vi "PH_BL-Master.Set Objects RC.vi"(0 "VI in":refnum<vi>, 1 "Boolean Status Service Subscriber before":T4(array[cluster]) {"Status" items=["no info", "off/false/out", "on/true/in", "Failure", "Alarm", "Status 1", "Status 2", "Status 3"]}, 2 "Picture Status Service Subscriber before":T4(array[cluster]) {"Status" items=["no info", "off/false/out", "on/true/in", "Failure", "Alarm", "Status 1", "Status 2", "Status 3"]}, 3 "Vacua before":T1(array[cluster]), 5 "error in (no error)":errorcluster) -> (14 "VI out":refnum<vi>, 19 "error out":errorcluster)   [LabVIEW 2014, in "PH_BL-Master.lvlib"]
uses:
  PH_BL-Master.lvlib
  PH_StatusHandler/PH_StatusHandler.Status.ctl
  PH_BL-Master.Status Subscriber Class.ctl
  PH_VacuumControl/PH_VacuumControl.lvlib
  PH_Common/PH_Common.lvlib
  PH_StatusHandler/PH_StatusHandler.lvlib
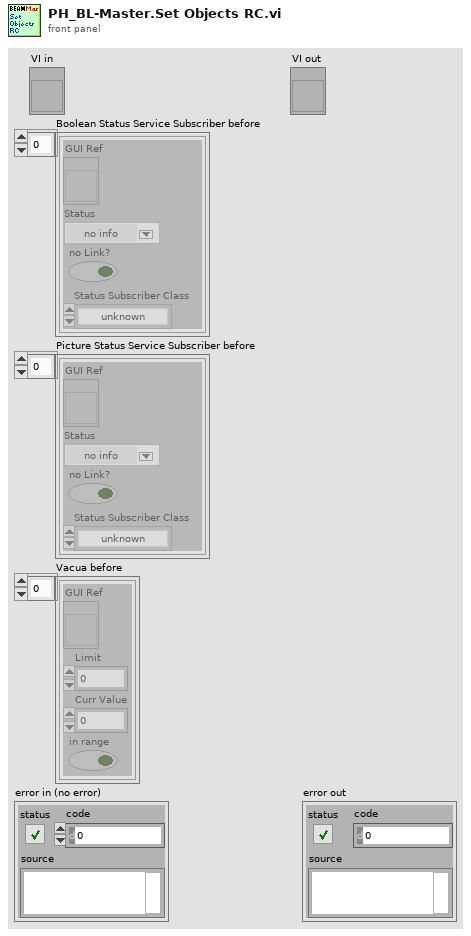
[diagram p1: front panel]
types:
  T1 = cluster{"GUI Ref":refnum<vi>, "Limit":dbl, "Curr Value":dbl, "in range":bool}[]
  T2 = typedef "PH_StatusHandler.lvlib/PH_StatusHandler.Status.ctl" = i16
  T3 = typedef "PH_BL-Master.lvlib/PH_BL-Master.Status Subscriber Class.ctl" = enum16{"unknown", "Switch", "BB", "6P Switch", "Switch GUI", "Switch and 6P State", "Force Sensor"}
  T4 = cluster{"GUI Ref":refnum<vi>, "Status":T2, "no Link?":bool, "Status Subscriber Class":T3}[]
  T5 = typedef "PH_BL-Master.lvlib/PH_BL-Master.i attribute.ctl" = cluster{"Remote controlled":bool, "Boolean Condition Service Subscriber":refnum<vi>[], "Picture Condition Service Subscriber":refnum<vi>[], "R2S":cluster{"GUI Ref":refnum<vi>, "State":bool}, "Vacua":cluster{"GUI Ref":refnum<vi>, "Limit":dbl, "Curr Value":dbl, "in range":bool}[], "O2 Inspection":cluster{"GUI Ref":refnum<vi>, "Concentration":dbl, "State":T2}[], "Boolean Status Service Subscriber":cluster{"GUI Ref":refnum<vi>, "Status":T2, "no Link?":bool, "Status Subscriber Class":T3}[], "Picture Status Service Subscriber":cluster{"GUI Ref":refnum<vi>, "Status":T2, "no Link?":bool, "Status Subscriber Class":T3}[], "6P 4Q Service Subscriber":cluster{"GUI Ref":refnum<vi>, "Selector":T6, "no Link?":bool}[], "Index of latest 6P 4Q changing Instance":i32, "Index of latest Picture Status changing Instance":i32, "Index of latest Boolean Status changing Instance":i32, "Vision ID on same Node":string, "Start Phase over?":bool, "GUI Ref Delete":refnum<vi>}
  T6 = typedef "PH_4_Pos_Selector.lvlib/PH_4_Pos_Selector.Position Selector.ctl" = u16
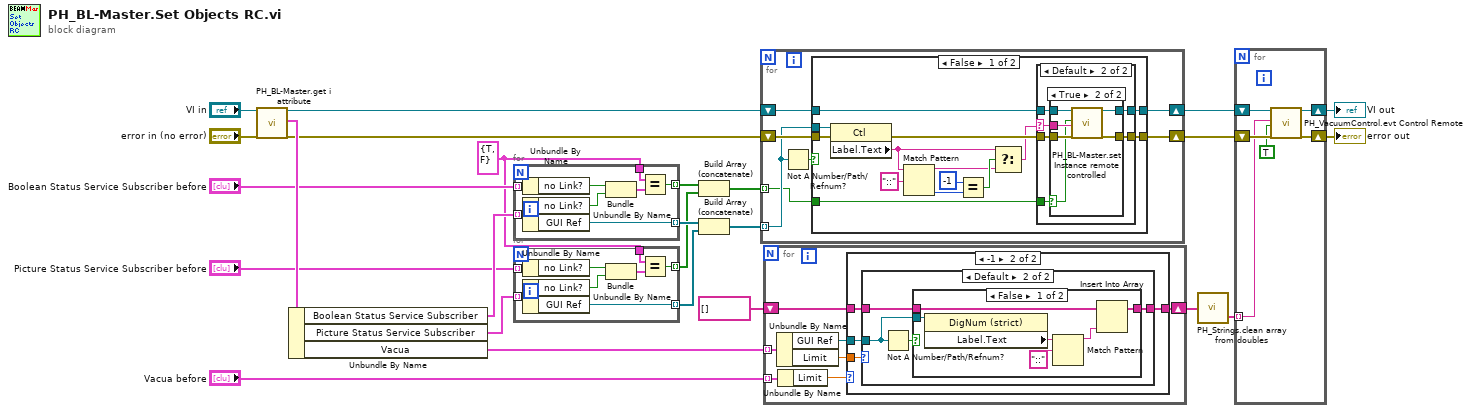
[diagram p0: block diagram]
diagram:
  w6 = cluster{"linked?":bool, "linked?":bool} {"linked?"=TRUE, "linked?"=FALSE} ("x")
  n1 = call "PH_BL-Master.get i attribute.vi"("i ref in"="VI in", "error in (no error)"="error in (no error)") -> ("i ref out"=w17:refnum<vi>, "i attribute"=w20:T5, "error out"=w19:errorcluster)  [unwired: 15 in]
  n2 = Unbundle By Name(w20) -> ("Boolean Status Service Subscriber"=w9:T4, "Picture Status Service Subscriber"=w2:T4, "Vacua"=w14:T1)
  n3 = for {
    tunnel: w9 -> [w33] mode=indexing
    tunnel: [w26] -> w8 mode=indexing
    tunnel: "Boolean Status Service Subscriber before" -> [w32] mode=indexing
    tunnel: w6 -> [w28]
    tunnel: [w27] -> w7 mode=indexing
    n4 = Unbundle By Name(w32) -> ("no Link?"=w31:bool)
    n5 = Unbundle By Name(w33) -> ("no Link?"=w30:bool, "GUI Ref"=w26:refnum<vi>)
    n6 = Bundle("no Link?"=w31, "no Link?"=w30) -> (w29:cluster{"no Link?":bool, "no Link?":bool})  [unwired: 1 in]
    n7 = Equal?(x=w28, y=w29) -> (x = y?=w27:bool)
  }
  n8 = for {
    tunnel: w2 -> [w41] mode=indexing
    tunnel: [w34] -> w5 mode=indexing
    tunnel: "Picture Status Service Subscriber before" -> [w40] mode=indexing
    tunnel: w6 -> [w36]
    tunnel: [w35] -> w4 mode=indexing
    n9 = Unbundle By Name(w40) -> ("no Link?"=w39:bool)
    n10 = Unbundle By Name(w41) -> ("no Link?"=w38:bool, "GUI Ref"=w34:refnum<vi>)
    n11 = Bundle("no Link?"=w39, "no Link?"=w38) -> (w37:cluster{"no Link?":bool, "no Link?":bool})  [unwired: 1 in]
    n12 = Equal?(x=w36, y=w37) -> (x = y?=w35:bool)
  }
  n13 = Build Array (concatenate)(w7, w4) -> (w11:bool[])
  n14 = Build Array (concatenate)(w8, w5) -> (w15:refnum<vi>[])
  n15 = for {
    shift-right: [w46] -> w21
    shift-left: w17 -> [w47]
    shift-right: [w45] -> w22
    shift-left: w19 -> [w48]
    tunnel: w15 -> [w43] mode=indexing
    tunnel: w11 -> [w42] mode=indexing
    n16 = Not A Number/Path/Refnum?(number/path/refnum=w43) -> (NaN/Path/Refnum?=w44:bool)
    n17 = case shown="False" w44 {
      tunnel: w48 -> [w62 w79]
      tunnel: w47 -> [w61 w80]
      tunnel: [w60 w80] -> w46
      tunnel: [w59 w79] -> w45
      tunnel: w43 -> [w57 _]
      tunnel: w42 -> [w50 _]
      frame False {
        n18 = property class="Ctl"(reference=w57, error in=w62) -> (error out=w58:errorcluster, "Label.Text"=w52:string)  [unwired: 1 out]
        n19 = Match Pattern(string=w52, regular expression="::") -> (before substring=w51:string, offset past match=w55:i32)  [unwired: 1 in, 2 out]
        n20 = Equal?(x=-1, y=w55) -> (x = y?=w53:bool)
        n21 = Select(t=w52, s=w53, f=w51) -> (s? t:f=w49:string)
        n22 = case shown="Default" w49 {
          selector: w49 -> [_ w65]
          tunnel: w61 -> [w64 w70]
          tunnel: [w64 w69] -> w60
          tunnel: [w63 w68] -> w59
          tunnel: w58 -> [w63 w67]
          tunnel: w50 -> [_ w66]
          frame "Shutter_Exp_Laserbay_Interlock", "Shutter_Laserlab_Interlock" {
          }
          frame Default {
            n23 = case shown="True" w66 {
              selector: w66 -> [_ w73]
              tunnel: w67 -> [w71 w78]
              tunnel: w70 -> [w72 w77]
              tunnel: [w72 w76] -> w69
              tunnel: [w71 w75] -> w68
              tunnel: w65 -> [_ w74]
              frame False {
              }
              frame True {
                n24 = call "PH_BL-Master.set Instance remote controlled.vi"("i ref in"=w77, "Remote Controlled (false)"=w73, "Instance Name"=w74, "error in"=w78) -> ("i ref out"=w76:refnum<vi>, "error out"=w75:errorcluster)  [unwired: 14 in]
              }
            }
          }
        }
      }
      frame True {
      }
    }
  }
  n25 = for {
    tunnel: w14 -> [w87] mode=indexing
    shift-right: [w85] -> w23
    shift-left: string[] [] -> [w84]
    tunnel: "Vacua before" -> [w82] mode=indexing
    n26 = Unbundle By Name(w87) -> ("GUI Ref"=w86:refnum<vi>, "Limit"=w83:dbl)
    n27 = Unbundle By Name(w82) -> ("Limit"=w81:dbl)
    n28 = case shown="-1" w81 {
      tunnel: w86 -> [_ w92]
      tunnel: [w88 w91] -> w85
      tunnel: w84 -> [w88 w90]
      tunnel: w83 -> [_ w89]
      frame 0, Default {
      }
      frame -1 {
        n29 = case shown="Default" w89 {
          tunnel: w92 -> [_ w96]
          tunnel: [w93 w95] -> w91
          tunnel: w90 -> [w93 w94]
          frame -1 {
          }
          frame Default {
            n30 = Not A Number/Path/Refnum?(number/path/refnum=w96) -> (NaN/Path/Refnum?=w97:bool)
            n31 = case shown="False" w97 {
              tunnel: w96 -> [w103 _]
              tunnel: [w100 w104] -> w95
              tunnel: w94 -> [w99 w104]
              frame False {
                n32 = property class="DigNum (strict)"(reference=w103) -> ("Label.Text"=w101:string)  [unwired: 1 in, 2 out]
                n33 = Match Pattern(string=w101, regular expression="::") -> (before substring=w98:string)  [unwired: 1 in, 3 out]
                n34 = Insert Into Array(array=w99, new element=w98) -> (w100:string[])  [unwired: 1 in]
              }
              frame True {
              }
            }
          }
        }
      }
    }
  }
  n35 = call "PH_Strings.clean array from doubles.vi"("Array Input"=w23) -> ("Cleaned Array Output"=w25:string[])  [unwired: 1 out]
  n36 = for {
    shift-right: [w109] -> w12
    shift-left: w21 -> [w110]
    shift-right: [w107] -> w13
    shift-left: w22 -> [w108]
    tunnel: w25 -> [w106] mode=indexing
    n37 = call "PH_VacuumControl.evt Control Remote.vi"("i ref in"=w110, "Instance"=w106, "Control Remote?"=TRUE, "error in (no error)"=w108) -> ("i ref out"=w109:refnum<vi>, "error out"=w107:errorcluster)  [unwired: 14 in]
  }
  "error out" <- w13
  "VI out" <- w12
